vi "SolidColor SetControl.vi"(0 "DeviceReference":T1, 1 "LEDStartIndex":i32, 2 "LEDEndIndex":i32, 3 "Color":i32, 7 "error in":errorcluster, 18 "Update Frequency (Hz)":dbl=100.0) -> (20 "DeviceReference Out":T1, 27 "error out":errorcluster)   [LabVIEW 2025]
doc: "Sets LEDs to a solid color."
uses:
  <vilib>/Rock Robotics/WPI/ThirdParty/Phoenix6/DeviceReference.ctl
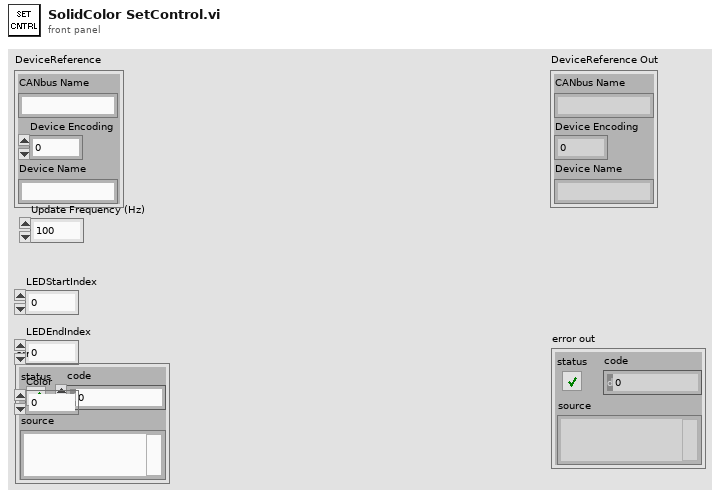
[diagram p1: front panel]
types:
  T1 = typedef "DeviceReference.ctl" = cluster{"CANbus Name":string, "Device Encoding":u32, "Device Name":string}
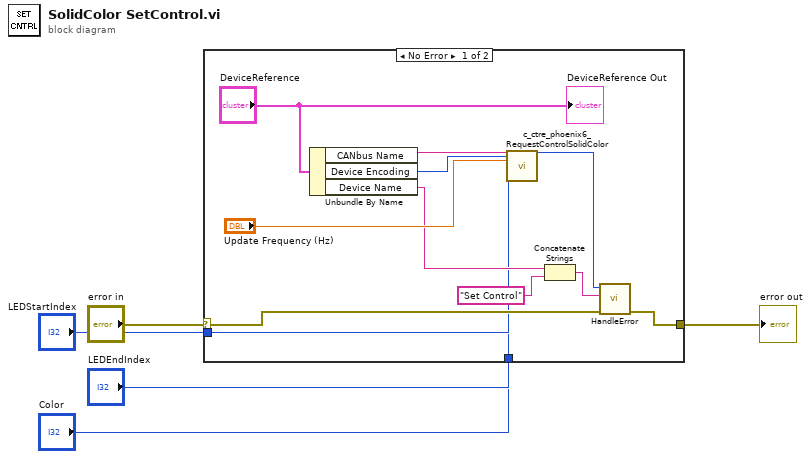
[diagram p0: block diagram]
diagram:
  n1 = case shown="No Error" "error in" {
    selector: "error in" -> [w13 w19]
    tunnel: [w12 w19] -> w4
    tunnel: "LEDStartIndex" -> [w8 _]
    tunnel: "LEDEndIndex" -> [w7 _]
    tunnel: "Color" -> [w6 _]
    frame No Error {
      n2 = Unbundle By Name("DeviceReference") -> ("CANbus Name"=w17:string, "Device Encoding"=w16:u32, "Device Name"=w11:string)
      n3 = call <vilib>:"c_ctre_phoenix6_RequestControlSolidColor.vi"("String 2"=w17, "Numeric 2"=w16, "Numeric 3"="Update Frequency (Hz)", "Numeric 4"=w8, "Numeric 5"=w7, "Numeric 6"=w6) -> ("Numeric"=w14:i32)  [unwired: 20 in, 1 out]
      n4 = Concatenate Strings(w11, "Set Control" ("origin")) -> (w9:string)
      n5 = call <vilib>:"HandleError.vi"("error in"=w13, "origin"=w9, "Status"=w14) -> ("error out"=w12:errorcluster)  [unwired: 8 in]
      "DeviceReference Out" <- "DeviceReference"
    }
    frame Error {
    }
  }
  "error out" <- w4
